vi "Get Subpanel VI Names.vi"(8 "error in (no error)":errorcluster, 11 "VI Panel Layout in":refnum<class "VI Panel Layout.lvclass">) -> (0 "error out":errorcluster, 1 "subpanel object UIDs":i32[](array[numeric]), 2 "VI names":string[](array[string]), 3 "VI Panel Layout out":refnum<class "VI Panel Layout.lvclass">, 4 "VI rel paths":path[](array[path]))   [LabVIEW 2010, in "NI_SE_Front Panel Layout.lvlib" / "VI Panel Layout.lvclass"]
uses:
  VI Panel Layout.lvclass
  VI Panel Layout.lvclass/VI Panel Layout.ctl
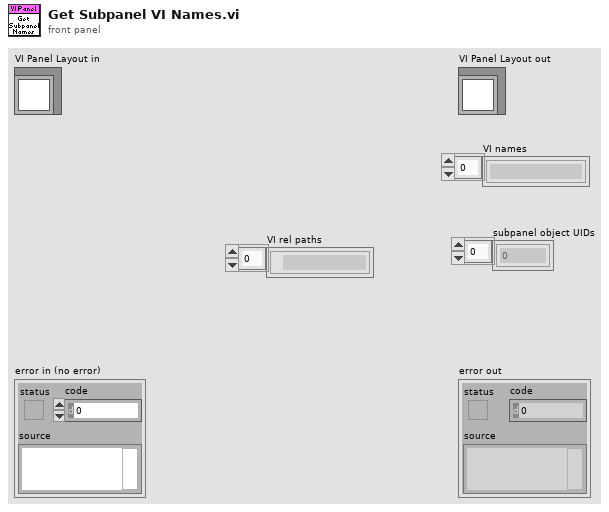
[diagram p1: front panel]
types:
  T1 = typedef "NI_SE_Front Panel Layout.lvlib/VI Panel Layout.lvclass/Subpanel VI Pair.ctl" = cluster{"subpanel UID":i32, "VI name":string, "VI path (rel)":path}
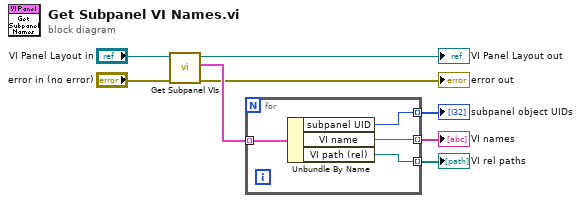
[diagram p0: block diagram]
diagram:
  n1 = call "Get Subpanel VIs.vi"("error in (no error)"="error in (no error)", "VI Panel Layout in"="VI Panel Layout in") -> ("error out"=→"error out":errorcluster, "subpanel VIs"=w5:T1[], "VI Panel Layout out"=→"VI Panel Layout out":refnum<class "VI Panel Layout.lvclass">)  [unwired: 7 in]
  n2 = for {
    tunnel: w5 -> [w12] mode=indexing
    tunnel: [w11] -> w4 mode=indexing
    tunnel: [w10] -> w2 mode=indexing
    tunnel: [w9] -> w1 mode=indexing
    n3 = Unbundle By Name(w12) -> ("subpanel UID"=w10:i32, "VI name"=w11:string, "VI path (rel)"=w9:path)
  }
  "VI names" <- w4
  "subpanel object UIDs" <- w2
  "VI rel paths" <- w1
